vi "AskInternet.vi"(11 "Message Received":string) -> (3 "body":string)   [LabVIEW 2020]
uses:
  <vilib>/httpClient/PUTBuffer.vi
  <vilib>/httpClient/LabVIEWHTTPClient.lvlib
panel:
  out "value":T1
  out "headers":string
  in  "error in (no error)":errorcluster
  out "error out":errorcluster
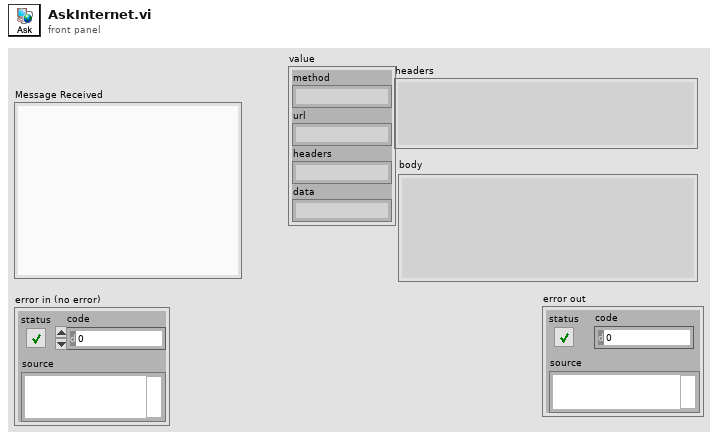
[diagram p1: front panel]
types:
  T1 = cluster{"method":string, "url":string, "headers":string, "data":string}
  T2 = typedef "LabVIEWHTTPClient.lvlib/ClientHandle.ctl" = refnum<k1>
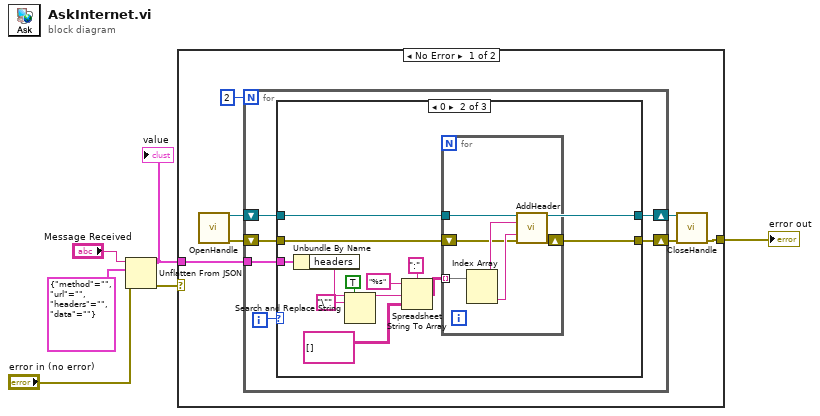
[diagram p0: block diagram]
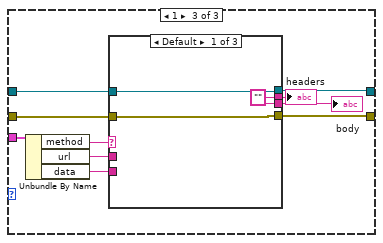
[diagram p3: hidden frame]
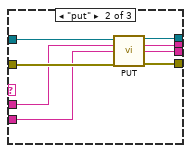
[diagram p4: hidden frame]
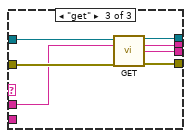
[diagram p5: hidden frame]
diagram:
  n1 = Unflatten From JSON(JSON string="Message Received", type and defaults=T1 {"method"="", "url"="", "headers"="", "data"=""}, error in (no error)="error in (no error)") -> (value=w3:T1, error out=w4:errorcluster)  [unwired: 4 in]
  "value" <- w3
  n2 = case shown="No Error" w4 {
    selector: w4 -> [_ w68]
    tunnel: w3 -> [w10 _]
    tunnel: [w7 w68] -> w2
    frame No Error {
      n3 = call <vilib>:"OpenHandle.vi"() -> ("client handle out"=w11:T2, "error out"=w12:errorcluster)  [unwired: 14 in]
      n4 = for {
        N: 2 -> [_]
        shift-right: [w18] -> w9
        shift-left: w11 -> [w17]
        shift-right: [w16] -> w8
        shift-left: w12 -> [w15]
        tunnel: w10 -> [w14]
        i -> [w19]
        n5 = case shown="0" w19 {
          tunnel: [w21 w25 w45] -> w18
          tunnel: w17 -> [w21 w25 w47]
          tunnel: [w20 w22 w44] -> w16
          tunnel: w15 -> [w20 w23 w46]
          tunnel: w14 -> [_ w33 w49]
          frame Default {
          }
          frame 0 {
            n6 = Unbundle By Name(w33) -> ("headers"=w32:string)
            n7 = Search and Replace String(replace all?=TRUE ("replace all? (F)"), input string=w32, search string="\"") -> (result string=w29:string)  [unwired: 5 in, 3 out]
            n8 = Spreadsheet String To Array(delimiter (Tab)=":", format string="%s", spreadsheet string=w29, array type (2D Dbl)=string[][] []) -> (array=w24:string[][])
            n9 = for {
              tunnel: w25 -> [w39]
              tunnel: w24 -> [w38] mode=indexing
              shift-right: [w34] -> w22
              shift-left: w23 -> [w35]
              n10 = Index Array(array=w38) -> (element #1=w37:string, element #2=w36:string)  [unwired: 2 in]
              n11 = call <vilib>:"AddHeader.vi"("client handle"=w39, "header"=w37, "value"=w36, "error in (no error)"=w35) -> ("error out"=w34:errorcluster)  [unwired: 10 in, 1 out]
            }
          }
          frame 1 {
            n12 = Unbundle By Name(w49) -> ("method"=w48:string, "url"=w43:string, "data"=w42:string)
            n13 = case shown="Default" w48 {
              tunnel: w47 -> [w52 w60 w67]
              tunnel: w46 -> [w51 w59 w66]
              tunnel: [w52 w58 w65] -> w45
              tunnel: [w51 w57 w64] -> w44
              tunnel: w43 -> [_ w56 w63]
              tunnel: w42 -> [_ w55 _]
              tunnel: [w50 w54 w62] -> w41
              tunnel: [w50 w53 w61] -> w40
              frame Default {
                w50 = "" ("headers")
              }
              frame "put" {
                n14 = call-poly <vilib>:"PUT.vi"("client handle"=w60, "url"=w56, "buffer"=w55, "error in (no error)"=w59) -> ("client handle out"=w58:T2, "headers"=w54:string, "body"=w53:string, "error out"=w57:errorcluster)  [unwired: 8 in]
              }
              frame "get" {
                n15 = call <vilib>:"GET.vi"("client handle"=w67, "url"=w63, "error in (no error)"=w66) -> ("client handle out"=w65:T2, "headers"=w62:string, "body"=w61:string, "error out"=w64:errorcluster)  [unwired: 9 in]
              }
            }
            "headers" <- w41
            "body" <- w40
          }
        }
      }
      n16 = call <vilib>:"CloseHandle.vi"("client handle"=w9, "error in (no error)"=w8) -> ("error out"=w7:errorcluster)  [unwired: 13 in]
    }
    frame Error {
    }
  }
  "error out" <- w2
